vi "TXTHDR_write.vi"(8 "error in (no error)":errorcluster, 10 "TXTHDR":T1, 11 "refnum in":refnum<file>) -> (0 "error out":errorcluster, 3 "refnum out":refnum<file>)   [LabVIEW 2012]
uses:
  TTTR_data_headers/TXTHDR.ctl
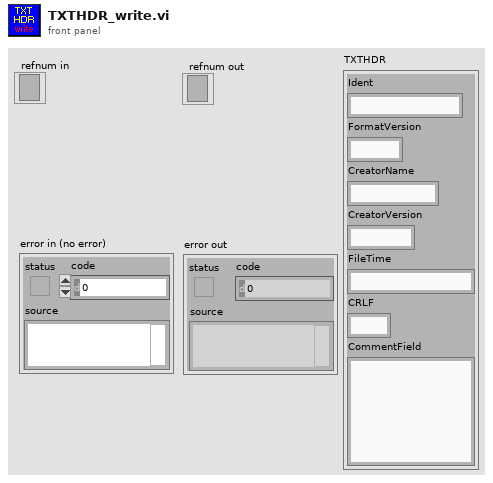
[diagram p1: front panel]
types:
  T1 = typedef "TXTHDR.ctl" = cluster{"Ident":string, "FormatVersion":string, "CreatorName":string, "CreatorVersion":string, "FileTime":string, "CRLF":string, "CommentField":string}
  T2 = enum16{"big-endian, network order", "native, host order", "little-endian"}
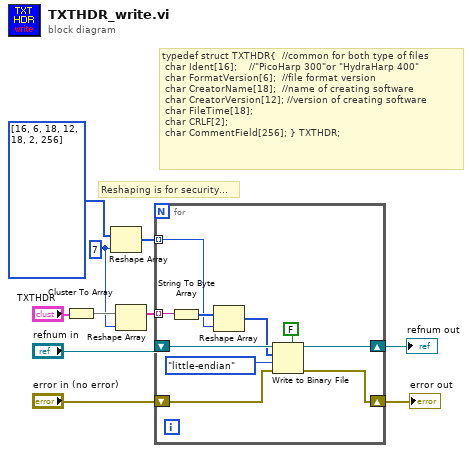
[diagram p0: block diagram]
diagram:
  w1 = 7
  # "Reshaping is for security..."
  # "typedef struct TXTHDR{\t\t//common for both type of files\n\tchar Ident[16];\t\t\t\t//\"PicoHarp 300\"or \"HydraHarp 400\"\n\tchar FormatVersion[6];\t\t//file format version\n\tchar CreatorName[18];\t\t//name of creating software\n\tchar CreatorVersion[12];\t//version of creating software\n\tchar FileTime[18];\n\tchar CRLF[2];\n\tchar CommentField[256]; } TXTHDR;"
  n1 = Cluster To Array(cluster="TXTHDR") -> (array=w3:string[])
  n2 = Reshape Array(i32[] [16, 6, 18, 12, 18, 2, 256], w1) -> (w4:i32[])
  n3 = Reshape Array(w3, w1) -> (w2:string[])
  n4 = for {
    tunnel: w4 -> [w13] mode=indexing
    shift-right: [w19] -> w8
    shift-left: "error in (no error)" -> [w20]
    shift-right: [w18] -> w6
    shift-left: "refnum in" -> [w17]
    tunnel: w2 -> [w15] mode=indexing
    n5 = String To Byte Array(string=w15) -> (unsigned byte array=w14:u8[])
    n6 = Reshape Array(w14, w13) -> (w12:u8[])
    n7 = Write to Binary File(file (use dialog)=w17, data=w12, error in=w20, 5:FALSE ("prepend array or string size? (T)"), 9:T2."little-endian" ("byte order (0:big-endian, network order)")) -> (refnum out=w18:refnum<file>, error out=w19:errorcluster)  [unwired: 1 in, 1 out]
  }
  "refnum out" <- w6
  "error out" <- w8
